vi "Shared Variable İzleme.vi"() -> ()   [LabVIEW 2014]
uses:
  CustomControls/TSE_Status.ctl
  CustomControls/Program_States.ctl
panel:
  out "OlcumNo":u16
  out "GKÇ-1_IP_Adresi":string
  out "TSE Status":T1={"Return Code"=0, "Message"="", "error in (no error)"={"status"=FALSE, "code"=0, "source"=""}, "Program State"=enum."Ön Yükleme Tamam", "Test A. Suresi"=0}
  out "GKÇ-1_Tipi":enum16{"", "PQ+", "PQ++", "ION"}(ring)
  out "GPIB_Interface_No":string
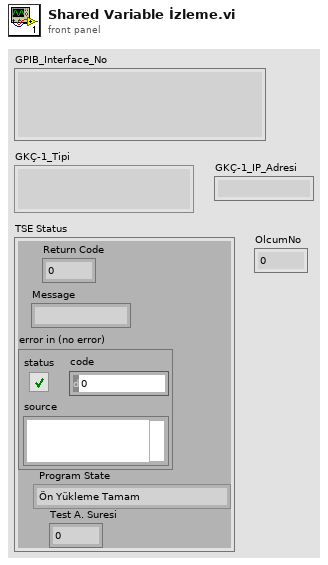
[diagram p1: front panel]
types:
  T1 = typedef "TSE_Status.ctl" = cluster{"Return Code":i32, "Message":string, "error in (no error)":errorcluster, "Program State":T2, "Test A. Suresi":u32}
  T2 = typedef "Program_States.ctl" = enum16{"Ön Yükleme", "TSE Baslat", "Kalibratöre Baglan", "Kalibratörü Baslat", "Ön Yükleme Tamam", "Frekans Testi", "Gerilim Testi", "Akim Testi", "Aktif Guc Testi", "Reaktif Guc Testi", "AC Akim Harmonik Testi", "AC Gerilim Harmonik Testi", "Flicker Testi", "Rapor Cikarma", "Yeniden Başlat", "Bekleme", "Durdur"}
  T3 = typedef "GKÇ_Tip.ctl" = enum16{"", "PQ+", "PQ++", "ION"}
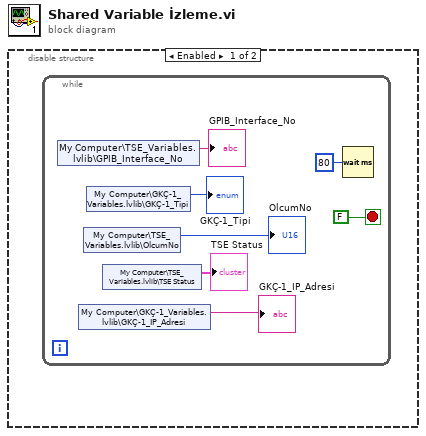
[diagram p0: block diagram]
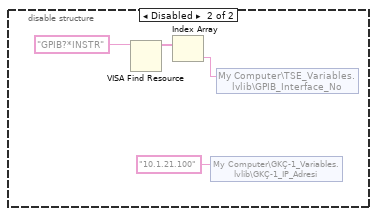
[diagram p2: hidden frame]
diagram:
  n1 = disable-structure shown="Enabled" {
    frame Enabled {
      n2 = while {
        stop <- FALSE stop-if-true
        n3 = shared-variable "My Computer\\TSE_Variables.lvlib\\GPIB_Interface_No"() -> (→"GPIB_Interface_No":string)  [unwired: 1 in, 1 out]
        n4 = shared-variable "My Computer\\GKÇ-1_Variables.lvlib\\GKÇ-1_IP_Adresi"() -> (→"GKÇ-1_IP_Adresi":string)  [unwired: 1 in, 1 out]
        n5 = shared-variable "My Computer\\TSE_Variables.lvlib\\OlcumNo"() -> (→"OlcumNo":u16)  [unwired: 1 in, 1 out]
        n6 = shared-variable "My Computer\\GKÇ-1_Variables.lvlib\\GKÇ-1_Tipi"() -> (→"GKÇ-1_Tipi":T3)  [unwired: 1 in, 1 out]
        n7 = shared-variable "My Computer\\TSE_Variables.lvlib\\TSE Status"() -> (→"TSE Status":T1)  [unwired: 1 in, 1 out]
        n8 = Wait (ms)(milliseconds to wait=u32 80) -> ()  [unwired: 1 out]
      }
    }
    frame Disabled {
      n9 = VISA Find Resource(11:"GPIB?*INSTR" ("expression (\"?*\")")) -> (3:w11:string[])  [unwired: 2 in, 2 out]
      n10 = Index Array(array=w11) -> (element=w9:string)  [unwired: 1 in]
      n11 = shared-variable "My Computer\\GKÇ-1_Variables.lvlib\\GKÇ-1_IP_Adresi"("10.1.21.100" ("GKÇ-1_IP_Adresi")) -> ()  [unwired: 1 in, 1 out]
      n12 = shared-variable "My Computer\\TSE_Variables.lvlib\\GPIB_Interface_No"(w9) -> ()  [unwired: 1 in, 1 out]
    }
  }
